vi "MeasureIV.vi"(5 "Junction Name":string, 6 "UiDefinition":T1, 7 ".NET Refnum":refnum<k24>, 8 "new file path (Not A Path if cancelled)":path, 9 "appended path":path, 11 ".NET Refnum in":refnum<k24>) -> (0 "error out":errorcluster)   [LabVIEW 2020]
uses:
  D:/LabviewDXFViewer/LabviewDXFViewer/bin/Release/LabviewDXFViewer.exe
  LabviewDXFViewer/bin/Release/LabviewDXFViewer.exe
  UIReferences.ctl
  <vilib>/Utility/file.llb/Write Delimited Spreadsheet (string).vi
  <vilib>/Utility/file.llb/Write Delimited Spreadsheet (DBL).vi
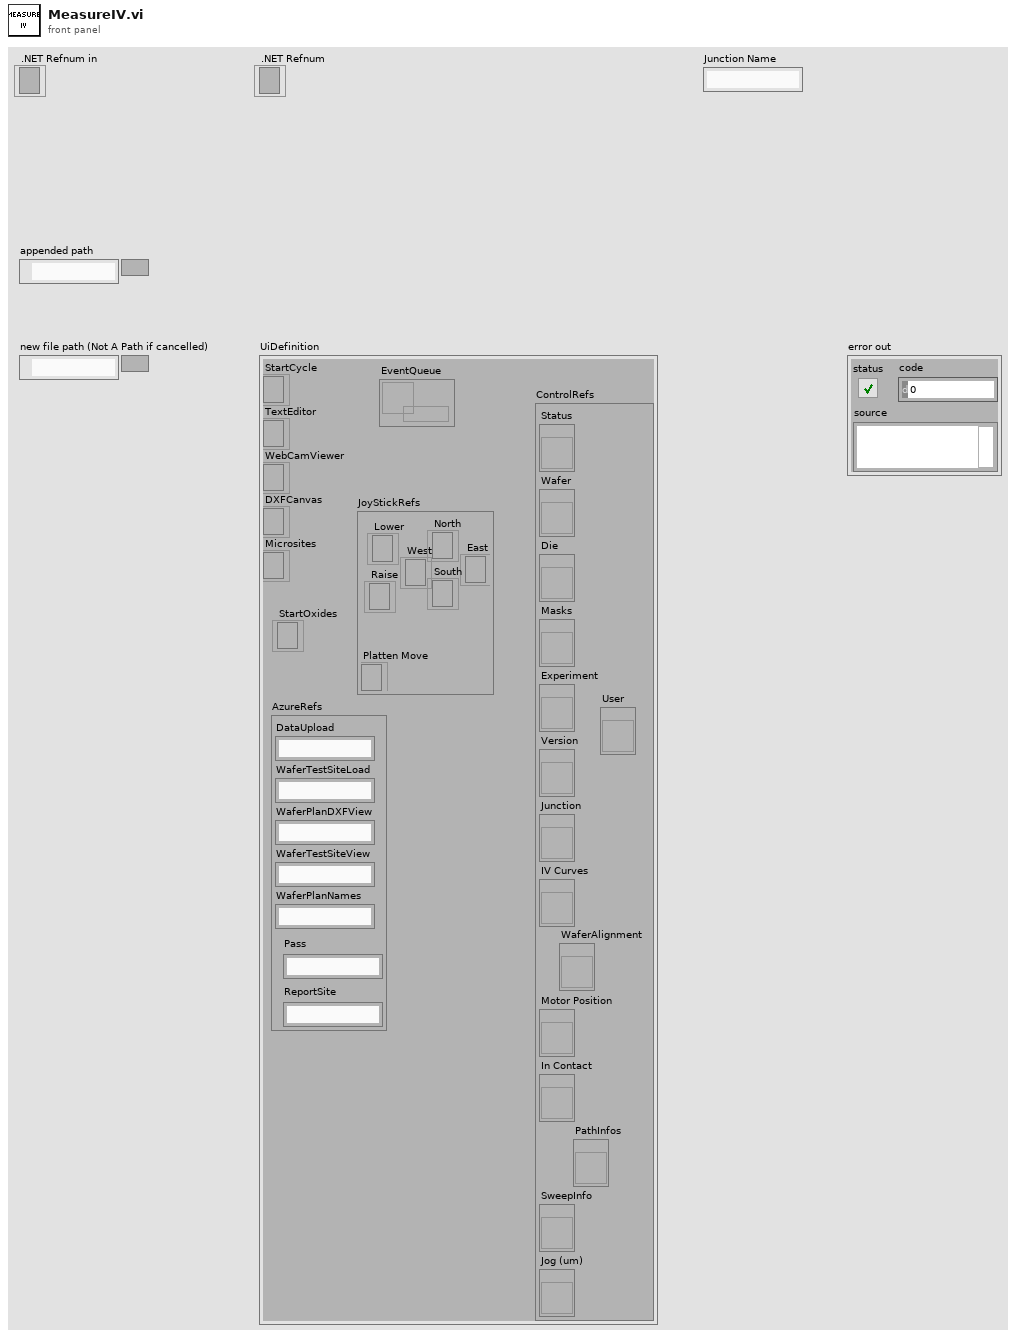
[diagram p1: front panel]
types:
  T1 = typedef "UIReferences.ctl" = cluster{"StartCycle":refnum<k24>, "TextEditor":refnum<k24>, "WebCamViewer":refnum<k24>, "DXFCanvas":refnum<k24>, "Microsites":refnum<k24>, "JoyStickRefs":cluster{"North":refnum<k24>, "Lower":refnum<k24>, "Raise":refnum<k24>, "Platten Move":refnum<k24>, "West":refnum<k24>, "East":refnum<k24>, "South":refnum<k24>}, "AzureRefs":cluster{"DataUpload":string, "WaferTestSiteLoad":string, "WaferPlanDXFView":string, "WaferTestSiteView":string, "WaferPlanNames":string, "Pass":string, "ReportSite":string}, "ControlRefs":cluster{"Status":refnum<vi>, "Wafer":refnum<vi>, "Die":refnum<vi>, "Masks":refnum<vi>, "Experiment":refnum<vi>, "Version":refnum<vi>, "Junction":refnum<vi>, "IV Curves":refnum<vi>, "Motor Position":refnum<vi>, "In Contact":refnum<vi>, "SweepInfo":refnum<vi>, "Jog (um)":refnum<vi>, "PathInfos":refnum<vi>, "User":refnum<vi>, "WaferAlignment":refnum<vi>}, "EventQueue":refnum<queue>, "StartOxides":refnum<k24>}
  T2 = typedef "CapacitanceInfos.ctl" = cluster{"Conductance":dbl, "CapacitanceIV":dbl, "Intercept":dbl, "CapacitanceSW":dbl, "Sum":dbl, "CapacitanceInfos":T3[], "CapacitancePhase":dbl, "dC/dV":dbl, "Function":string}
  T3 = typedef "CapacitanceRecord.ctl" = cluster{"Freq":dbl, "Vpp":dbl, "PhaseS":dbl, "Irms":dbl, "PhaseC":dbl, "Theta":dbl, "VDrive":dbl, "Capacitance":dbl, "Other":dbl}
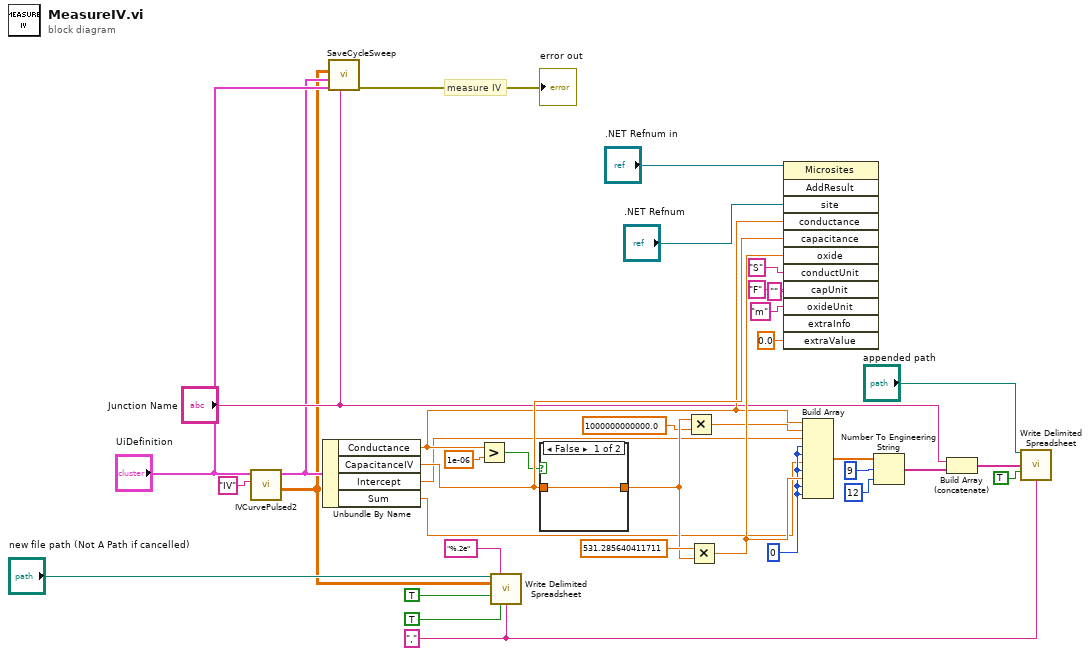
[diagram p0: block diagram]
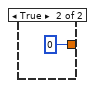
[diagram p2: hidden frame]
diagram:
  w4 = "," ("delimiter (\\t)")
  w32 = 0
  # "measure IV"
  n1 = call "IVCurvePulsed2.vi"("Program"="IV", "UiDefinition"="UiDefinition") -> ("appended array"=w12:dbl[][], "InfoCluster"=w25:T2)  [unwired: 8 in]
  n2 = Unbundle By Name(w25) -> ("Conductance"=w33:dbl, "CapacitanceIV"=w34:dbl, "Intercept"=w15:dbl, "Sum"=w16:dbl)
  n3 = call "SaveCycleSweep.vi"("JunctionName"="Junction Name", "UiDefinition 2"="UiDefinition", "InfoCluster"=w25, "appended array"=w12) -> ("error out"=→"error out":errorcluster)  [unwired: 7 in]
  n4 = Greater?(x=w33, y=1e-06) -> (0:w19:bool)
  n5 = call-poly <vilib>:"Write Delimited Spreadsheet.vi"("file path (dialog if empty)"="new file path (Not A Path if cancelled)", "format (%.3f)"="%.2e", "2D data"=w12, "append to file? (new file:F)"=TRUE, "transpose? (no:F)"=TRUE, "delimiter (\\t)"=w4) -> ()  [unwired: 8 in, 2 out]
  n6 = case shown="False" w19 {
    tunnel: [w38 0] -> w35
    tunnel: w34 -> [w38 _]
    frame False {
    }
    frame True {
    }
  }
  n7 = Multiply(x=w35, y=1000000000000.0) -> (x*y=w17:dbl)
  n8 = Multiply(x=531.285640411711, y=w35) -> (x*y=w37:dbl)
  n9 = invoke class="Microsites" method="AddResult"(reference=".NET Refnum in", "site"=".NET Refnum", "conductance"=w33, "capacitance"=w34, "oxide"=w37, "conductUnit"="S", "capUnit"="F", "oxideUnit"="m" ("interceptUnit"), "extraInfo"="", "extraValue"=0.0) -> ()  [unwired: 2 in, 12 out]
  n10 = Build Array(w33, w17, w15, w32, w32, w16, w32, w37, w32, w32) -> (w14:dbl[])
  n11 = Number To Engineering String(2:i16 12 ("precision (6)"), 3:i16 9 ("width (-)"), 4:w14) -> (0:w6:string[])  [unwired: 1 in]
  n12 = Build Array (concatenate)("Junction Name", w6) -> (w8:string[])
  n13 = call-poly <vilib>:"Write Delimited Spreadsheet.vi"("file path (dialog if empty)"="appended path", "1D data"=w8, "append to file? (new file:F)"=TRUE, "delimiter (\\t)"=w4) -> ()  [unwired: 10 in, 2 out]
